vi "testcompile.vi"() -> ()   [LabVIEW 2013]
uses:
  <vilib>/Platform/TimedLoop/XDataNode/wakeup.ctl
  <vilib>/Platform/TimedLoop/XDataNode/XDNodeRunTimeDep.lvlib
  <vilib>/Platform/TimedLoop/XDataNode/nitl_modes.ctl
  <vilib>/Platform/TimedLoop/XDataNode/timing_clust.ctl
  <vilib>/Platform/TimedLoop/XDataNode/XDataNode.xnode
  <vilib>/rvi/DataTransferAndStorage/Container/XNode/niFpgaContainer.xnode
  <vilib>/rvi/FIFO/Fifo_Resource/nirvififoEmulationWrite.vi
  <vilib>/rvi/FIFO/Fifo_Resource/nirvififoEmulationRead.vi
  FPGA/Sector/Accumulate/Sector Parameter Cluster.ctl
panel:
  in  "Sector Parameters Left":T1={"Start Angle"=0.6541748046875, "End Angle"=0.856201171875, "Inner Radius"=309, "Outter Radius"=405, "Hinge X"=947, "Hinge Y"=829, "NumWingSectors"=8}
  in  "Sector Parameters Right":T1={"Start Angle"=0.13543701171875, "End Angle"=0.30462646484375, "Inner Radius"=309, "Outter Radius"=405, "Hinge X"=1106, "Hinge Y"=803, "NumWingSectors"=8}
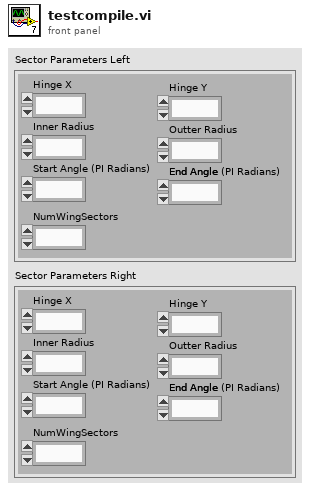
[diagram p1: front panel]
types:
  T1 = typedef "Sector Parameter Cluster.ctl" = cluster{"Start Angle":fxp<+,17,3>, "End Angle":fxp<+,17,3>, "Inner Radius":u16, "Outter Radius":u16, "Hinge X":u16, "Hinge Y":u16, "NumWingSectors":u8}
  T2 = typedef "XDNodeRunTimeDep.lvlib/timing_clust.ctl" = cluster{"Expected End [f-1]":u64, "Actual End [f-1]":u64, "Finished Late? [f-1]":bool, "Expected End [i-1]":u64, "Actual End [i-1]":u64, "Finished Late? [i-1]":bool, "Expected Start [i]":u64, "Actual Start [i]":u64, "Expected Start [f]":u64, "Actual Start [f]":u64, "Source Name":string, "Structure Name":string, "Period":i64, "Deadline":i64, "Offset":i64, "Start":i64, "Priority":i32, "Timeout":i32, "Mode":T3, "Wakeup Reason":T4, "Error":errorcluster, "Source Type":string, "Secondary Source Type":string, "Global End Time":u64, "Global Start Time":u64, "Frame Duration":u64, "Iteration Duration":u64, "Assigned CPU":i32, "I/O Scan Engine Mode":u32}
  T3 = typedef "XDNodeRunTimeDep.lvlib/nitl_modes.ctl" = enum32{"No Change", "Process missed periods, maintain original phase", "Discard missed periods, maintain original phase", "Process missed periods, ignore original phase", "Discard missed periods, ignore original phase"}
  T4 = typedef "XDNodeRunTimeDep.lvlib/wakeup.ctl" = enum32{"Normal", "Aborted", "Asynchronous wakeup", "Timing source error", "Timed loop error", "Timeout"}
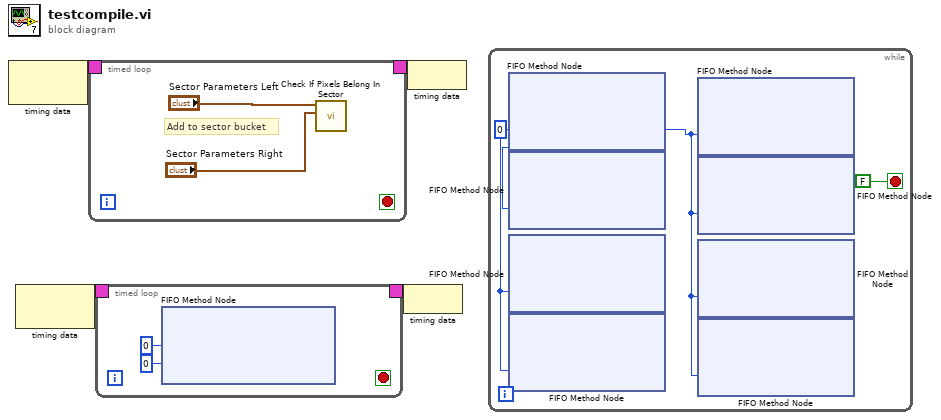
[diagram p0: block diagram]
diagram:
  n1 = node-c288() -> (w4:T2)  [unwired: 1 in]
  n2 = node-c288() -> (w2:T2)  [unwired: 1 in]
  n3 = timed-loop {
    timing: w4 -> [_]
    timing-out: [_] -> w3
    stop <- _ stop-if-true
    # "Add to sector bucket"
    n4 = call "Check If Pixels Belong In Sector.vi"("Sector Parameters Right"="Sector Parameters Right", "Sector Parameters Left"="Sector Parameters Left") -> ()  [unwired: 9 in, 1 out]
  }
  n5 = timed-loop {
    timing: w2 -> [_]
    timing-out: [_] -> w1
    stop <- _ stop-if-true
    n6 = xnode ("FIFO Method Node")("Element"=u64 0, "Timeout"=0) -> ()  [unwired: 1 in, 2 out]
  }
  n7 = node-c288(w1) -> ()
  n8 = node-c288(w3) -> ()
  n9 = while {
    stop <- FALSE stop-if-true
    w13 = 0 ("Timeout")
    n10 = xnode ("FIFO Method Node")("Timeout"=w13) -> ()  [unwired: 1 in, 3 out]
    n11 = xnode ("FIFO Method Node")("Timeout"=w13) -> ()  [unwired: 1 in, 3 out]
    n12 = xnode ("FIFO Method Node")("Timeout"=w13) -> ()  [unwired: 1 in, 3 out]
    n13 = xnode ("FIFO Method Node")("Timeout"=w13) -> ()  [unwired: 1 in, 3 out]
    n14 = xnode ("FIFO Method Node")("Timeout"=w13) -> ()  [unwired: 1 in, 3 out]
    n15 = xnode ("FIFO Method Node")("Timeout"=w13) -> ()  [unwired: 1 in, 3 out]
    n16 = xnode ("FIFO Method Node")("Timeout"=w13) -> ()  [unwired: 1 in, 3 out]
    n17 = xnode ("FIFO Method Node")("Timeout"=w13) -> ()  [unwired: 1 in, 3 out]
  }
